vi "DayNight_check.vi"() -> (1 "Day?":bool)   [LabVIEW 2020]
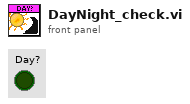
[diagram p1: front panel]
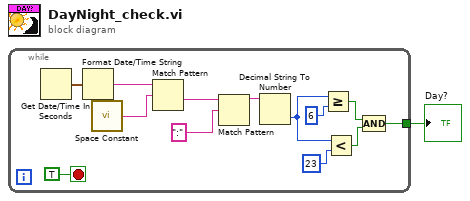
[diagram p0: block diagram]
diagram:
  n1 = while {
    tunnel: [w12] -> w1
    stop <- TRUE stop-if-true
    n2 = Get Date/Time In Seconds() -> (seconds since 1Jan1904=w6:timestamp)
    n3 = Format Date/Time String(seconds (now)=w6) -> (date/time string=w7:string)  [unwired: 2 in]
    n4 = call <vilib>:"Space Constant.vi"() -> ("String"=w8:string)
    n5 = Match Pattern(string=w7, regular expression=w8) -> (after substring=w9:string)  [unwired: 1 in, 3 out]
    n6 = Match Pattern(string=w9, regular expression=":") -> (before substring=w10:string)  [unwired: 1 in, 3 out]
    n7 = Decimal String To Number(string=w10) -> (number=w4:i32)  [unwired: 2 in, 1 out]
    n8 = Greater Or Equal?(x=w4, y=6) -> (x >= y?=w14:bool)
    n9 = Less?(x=w4, y=23) -> (x < y?=w13:bool)
    n10 = Compound Arithmetic op=AND(w14, w13) -> (w12:bool)
  }
  "Day?" <- w1
